vi "输入密码对话框.vi"() -> (3 "密码正确":bool)   [LabVIEW 2014]
panel:
  in  "取消按钮":bool
  in  "确定按钮":bool
  in  "请输入密码":string
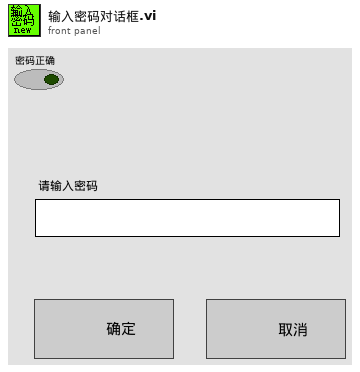
[diagram p1: front panel]
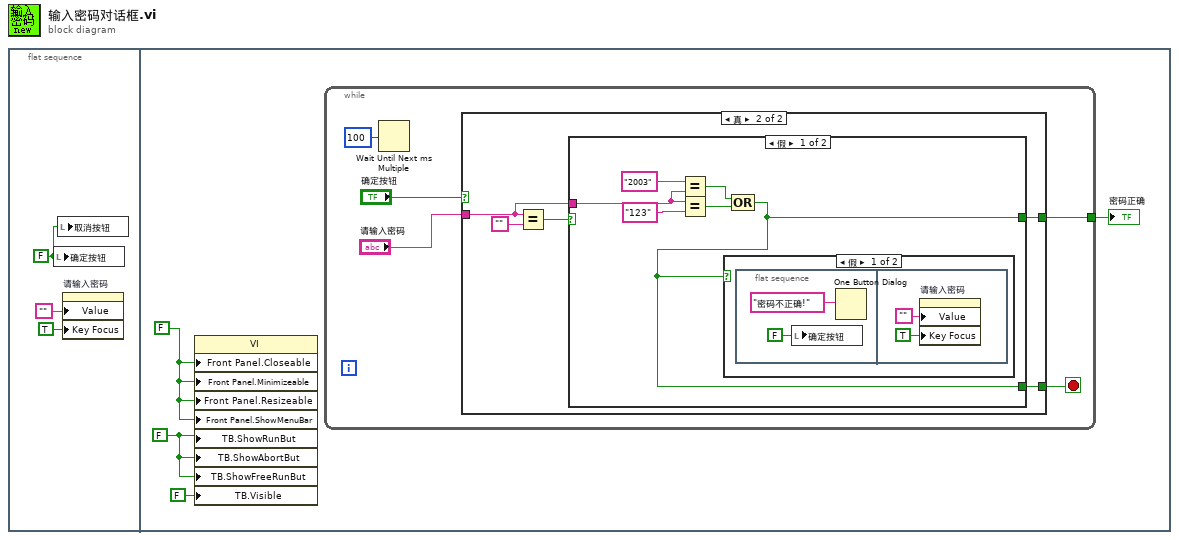
[diagram p0: block diagram]
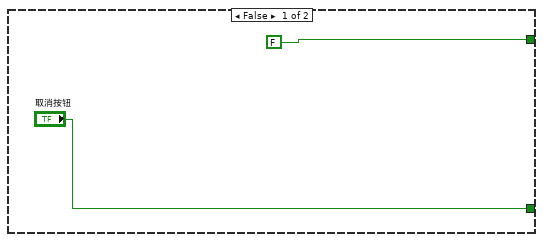
[diagram p2: hidden frame]
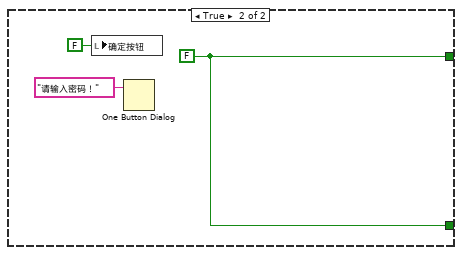
[diagram p4: hidden frame]
diagram:
  n1 = flat-sequence {
    frame #0 {
      w2 = FALSE ("确定按钮")
      n2 = local write "确定按钮"(w2) -> ()
      n3 = local write "取消按钮"(w2) -> ()
      n4 = property on="请输入密码" class="Str"("Value"="" ("请输入密码"), "Key Focus"=TRUE ("键选中")) -> ()  [unwired: 2 in, 2 out]
    }
    frame #1 {
      w5 = FALSE ("Front Panel Window:Closeable")
      w7 = FALSE ("Front Panel Window:Closeable")
      n5 = property class="VI"("Front Panel.Closeable"=w7, "Front Panel.Minimizeable"=w7, "Front Panel.Resizeable"=w7, "Front Panel.ShowMenuBar"=w7, "TB.ShowRunBut"=w5, "TB.ShowAbortBut"=w5, "TB.ShowFreeRunBut"=w5, "TB.Visible"=FALSE ("工具栏:可见")) -> ()  [unwired: 2 in, 2 out]
      n6 = while {
        tunnel: [w8] -> w6
        stop <- w11 stop-if-true
        n7 = Wait Until Next ms Multiple(millisecond multiple=i64 100 ("Period")) -> ()  [unwired: 1 out]
        n8 = case shown="真" "确定按钮" {
          tunnel: ["取消按钮" w16] -> w11
          tunnel: "请输入密码" -> [_ w18]
          tunnel: [FALSE w17] -> w8
          frame False {
          }
          frame True {
            n9 = Equal?(x=w18, y="") -> (x = y?=w15:bool)
            n10 = case shown="假" w15 {
              tunnel: w18 -> [w23 _]
              tunnel: [w20 w30] -> w17
              tunnel: [w20 w30] -> w16
              frame False {
                n11 = Equal?(x="2003", y=w23) -> (x = y?=w21:bool)
                n12 = Equal?(x=w23, y="123") -> (x = y?=w24:bool)
                n13 = Compound Arithmetic op=OR(w21, w24) -> (w20:bool)
                n14 = case shown="假" w20 {
                  frame False {
                    n15 = flat-sequence {
                      frame #0 {
                        n16 = local write "确定按钮"(FALSE ("确定按钮")) -> ()
                        n17 = One Button Dialog(message="密码不正确!" ("y")) -> ()  [unwired: 1 in, 1 out]
                      }
                      frame #1 {
                        n18 = property on="请输入密码" class="Str"("Value"="" ("请输入密码"), "Key Focus"=TRUE ("键选中")) -> ()  [unwired: 2 in, 2 out]
                      }
                    }
                  }
                  frame True {
                  }
                }
              }
              frame True {
                w30 = FALSE
                n19 = local write "确定按钮"(FALSE ("确定按钮")) -> ()
                n20 = One Button Dialog(message="请输入密码！" ("消息")) -> ()  [unwired: 1 in, 1 out]
              }
            }
          }
        }
      }
      "密码正确" <- w6
    }
  }
